vi "Scale Arbitrary Waveform.vi"(8 "error in (no error)":errorcluster, 10 "Arbitrary Waveform Data":dbl[](array[numeric]), 11 "VISA resource name":refnum<visa-resource-name>) -> (0 "error out":errorcluster, 2 "Scaled Arbitrary Waveform Data":i16[](array[numeric]), 3 "VISA resource name out":refnum<visa-resource-name>)   [LabVIEW 2023, in "Keysight-33500B.lvlib"]
doc: "Scales a data array so that the maximum (positive or negative) value in the array corresponds to the maximum allowed value (positive or negative) for the instrument."
uses:
  Keysight-33500B.lvlib
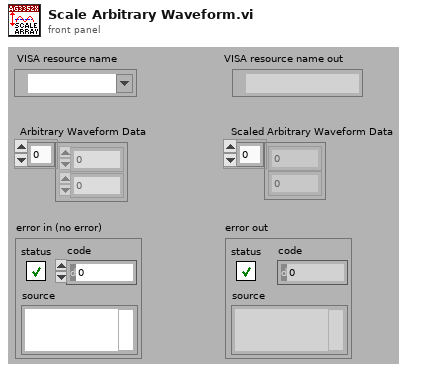
[diagram p1: front panel]
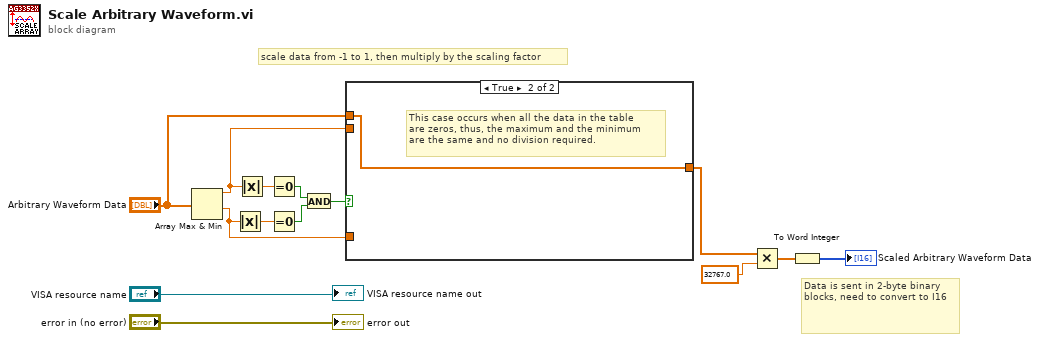
[diagram p0: block diagram]
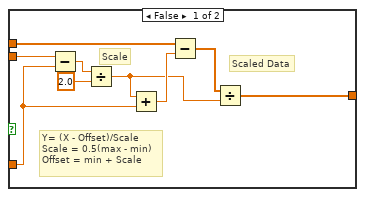
[diagram p2: hidden frame]
diagram:
  # "Data is sent in 2-byte binary blocks, need to convert to I16"
  # "scale data from -1 to 1, then multiply by the scaling factor"
  n1 = Array Max & Min(array="Arbitrary Waveform Data") -> (max value=w7:dbl, min value=w6:dbl)  [unwired: 2 out]
  n2 = Absolute Value(x=w6) -> (abs(x)=w10:dbl)
  n3 = Absolute Value(x=w7) -> (abs(x)=w9:dbl)
  n4 = Equal To 0?(x=w9) -> (x = 0?=w12:bool)
  n5 = Equal To 0?(x=w10) -> (x = 0?=w11:bool)
  n6 = And(x=w12, y=w11) -> (x .and. y?=w8:bool)
  n7 = case shown="True" w8 {
    tunnel: w6 -> [w20 _]
    tunnel: w7 -> [w23 _]
    tunnel: "Arbitrary Waveform Data" -> [w19 w24]
    tunnel: [w15 w24] -> w4
    frame False {
      # "Y= (X - Offset)/Scale\nScale = 0.5(max - min)\nOffset = min + Scale"
      # "Scale"
      # "Scaled Data"
      n8 = Subtract(x=w23, y=w20) -> (x-y=w22:dbl)
      n9 = Divide(x=w22, y=2.0) -> (x/y=w16:dbl)
      n10 = Add(x=w16, y=w20) -> (x+y=w18:dbl)
      n11 = Subtract(x=w19, y=w18) -> (x-y=w17:dbl[])
      n12 = Divide(x=w17, y=w16) -> (x/y=w15:dbl[])
    }
    frame True {
      # "This case occurs when all the data in the table\nare zeros, thus, the maximum and the minimum\nare the same and no division required."
    }
  }
  n13 = Multiply(x=w4, y=32767.0) -> (x*y=w13:dbl[])
  n14 = To Word Integer(number=w13) -> (16bit integer=→"Scaled Arbitrary Waveform Data":i16[])
  "VISA resource name out" <- "VISA resource name"
  "error out" <- "error in (no error)"
